vi "test-macro-menus.vi"   [LabVIEW 2019]
uses:
  <vilib>/Rock Robotics/WPI/ThirdParty/JAS_Junk/TrajLib/Trajectory_Library.lvlib
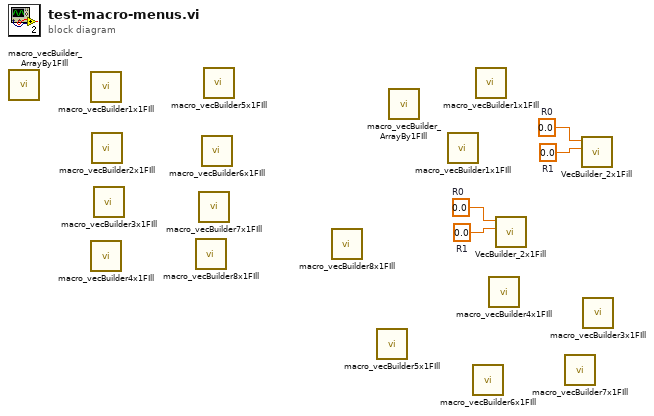
[diagram p0: block diagram]
diagram:
  w2 = 0.0  # R1
  w1 = 0.0  # R0
  w4 = 0.0  # R1
  w3 = 0.0  # R0
  n1 = call <vilib>:"macro_vecBuilder_ArrayBy1FIll.vi"() -> ()  [unwired: 12 in]
  n2 = call <vilib>:"macro_vecBuilder1x1FIll.vi"() -> ()  [unwired: 12 in]
  n3 = call <vilib>:"macro_vecBuilder4x1FIll.vi"() -> ()  [unwired: 12 in]
  n4 = call <vilib>:"macro_vecBuilder2x1FIll.vi"() -> ()  [unwired: 12 in]
  n5 = call <vilib>:"macro_vecBuilder3x1FIll.vi"() -> ()  [unwired: 12 in]
  n6 = call <vilib>:"macro_vecBuilder8x1FIll.vi"() -> ()  [unwired: 12 in]
  n7 = call <vilib>:"macro_vecBuilder7x1FIll.vi"() -> ()  [unwired: 12 in]
  n8 = call <vilib>:"macro_vecBuilder6x1FIll.vi"() -> ()  [unwired: 12 in]
  n9 = call <vilib>:"macro_vecBuilder5x1FIll.vi"() -> ()  [unwired: 12 in]
  n10 = call <vilib>:"macro_vecBuilder8x1FIll.vi"() -> ()  [unwired: 12 in]
  n11 = call <vilib>:"macro_vecBuilder5x1FIll.vi"() -> ()  [unwired: 12 in]
  n12 = call <vilib>:"macro_vecBuilder_ArrayBy1FIll.vi"() -> ()  [unwired: 12 in]
  n13 = call <vilib>:"macro_vecBuilder1x1FIll.vi"() -> ()  [unwired: 12 in]
  n14 = call <vilib>:"macro_vecBuilder6x1FIll.vi"() -> ()  [unwired: 12 in]
  n15 = call <vilib>:"macro_vecBuilder1x1FIll.vi"() -> ()  [unwired: 12 in]
  n16 = call <vilib>:"macro_vecBuilder4x1FIll.vi"() -> ()  [unwired: 12 in]
  n17 = call <vilib>:"VecBuilder_2x1Fill.vi"("R1"=w4, "R0"=w3) -> ()  [unwired: 9 in, 1 out]
  n18 = call <vilib>:"macro_vecBuilder7x1FIll.vi"() -> ()  [unwired: 12 in]
  n19 = call <vilib>:"VecBuilder_2x1Fill.vi"("R1"=w2, "R0"=w1) -> ()  [unwired: 9 in, 1 out]
  n20 = call <vilib>:"macro_vecBuilder3x1FIll.vi"() -> ()  [unwired: 12 in]
